vi "Get settings chain.vi"(8 "error in (no error)":errorcluster, 11 "ExampleClassB in":refnum<class "ExampleClassB.lvclass">) -> (0 "error out":errorcluster, 1 "class name":string[](array[string]), 2 "settings":variant[](array[variant]), 3 "ExampleClassB out":refnum<class "ExampleClassB.lvclass">)   [LabVIEW 2012, in "ExampleClassB.lvclass"]
doc: "Returns an array of variants containing the settings clusters of each class in the inheritance chain (lowest child class first), together with an array of all class names in the inheritance chain.\n\nFor classes without settings cluster, the settings chain contains empty variants."
uses:
  ExampleClassB.lvclass
  <vilib>/Distrio/Murmex/Murmex/Murmex.lvclass
  ExampleClassB.lvclass/ExampleClassB.ctl
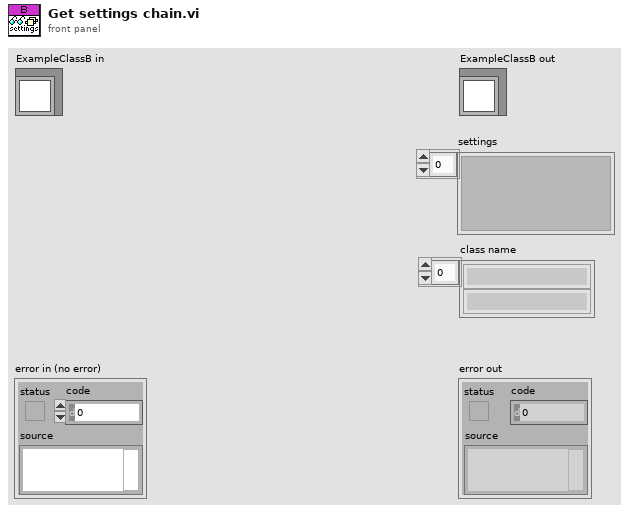
[diagram p1: front panel]
types:
  T1 = typedef "ExampleClassB.lvclass/Settings cluster.ctl" = cluster{"expected samples":i32}
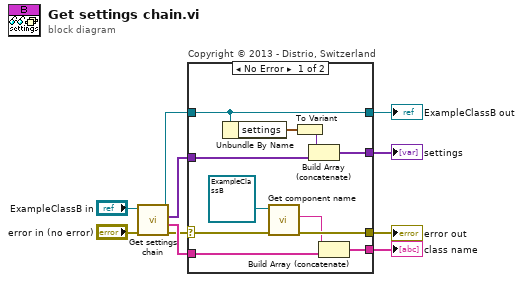
[diagram p0: block diagram]
diagram:
  n1 = call-parent "Get settings chain.vi"("error in (no error)"="error in (no error)", "MurmexBase in"="ExampleClassB in") -> ("error out"=w6:errorcluster, "class name"=w7:string[], "settings"=w8:variant[], "MurmexBase out"=w1:refnum<class "ExampleClassB.lvclass">)  [unwired: 6 in]
  n2 = case "Copyright © 2013 - Distrio, Switzerland" shown="No Error" w6 {
    selector: w6 -> [w20 w23]
    tunnel: [w21 w23] -> w5
    tunnel: [w18 _] -> w4
    tunnel: [w17 _] -> w3
    tunnel: [w12 w22] -> w2
    tunnel: w8 -> [w15 _]
    tunnel: w7 -> [w16 _]
    tunnel: w1 -> [w12 w22]
    frame No Error {
      n3 = Unbundle By Name(w12) -> ("settings"=w14:T1)
      n4 = call <vilib>:"Get component name.vi"("error in (no error)"=w20, "Murmex in"=refnum<class "ExampleClassB.lvclass"> refnum ("ExampleClassB in")) -> ("error out"=w21:errorcluster, "component name"=w19:string)  [unwired: 7 in, 1 out]
      n5 = To Variant(anything=w14) -> (Variant=w13:variant)
      n6 = Build Array (concatenate)(w13, w15) -> (w17:variant[])
      n7 = Build Array (concatenate)(w19, w16) -> (w18:string[])
    }
    frame Error {
    }
  }
  "error out" <- w5
  "ExampleClassB out" <- w2
  "settings" <- w3
  "class name" <- w4
